vi "Gui.TopBar.Setting.vi"(7 "pane ref in":refnum<vi>, 8 "error in":errorcluster, 9 "values":T1={"OK"=FALSE, "Cancel"=FALSE, "Reload"=FALSE, "Save"=FALSE, "Module name"="NAME"}, 10 "visibility":T6, 11 "top bar ref in":refnum<vi>) -> (0 "error out":errorcluster, 3 "top bar ref out":refnum<vi>)   [LabVIEW 2019, in "Main.lvlib"]
uses:
  Main.lvlib
  Gui.TopBar.Visibility.ctl
  Gui.TopBar.ctl
  Framework/Tools/controls/buttons/OK.ctl
  Framework/Tools/controls/buttons/Cancel.ctl
  Framework/Tools/controls/buttons/Reload.ctl
  Framework/Tools/controls/buttons/Save.ctl
  Framework/Tools/Tools.lvlib
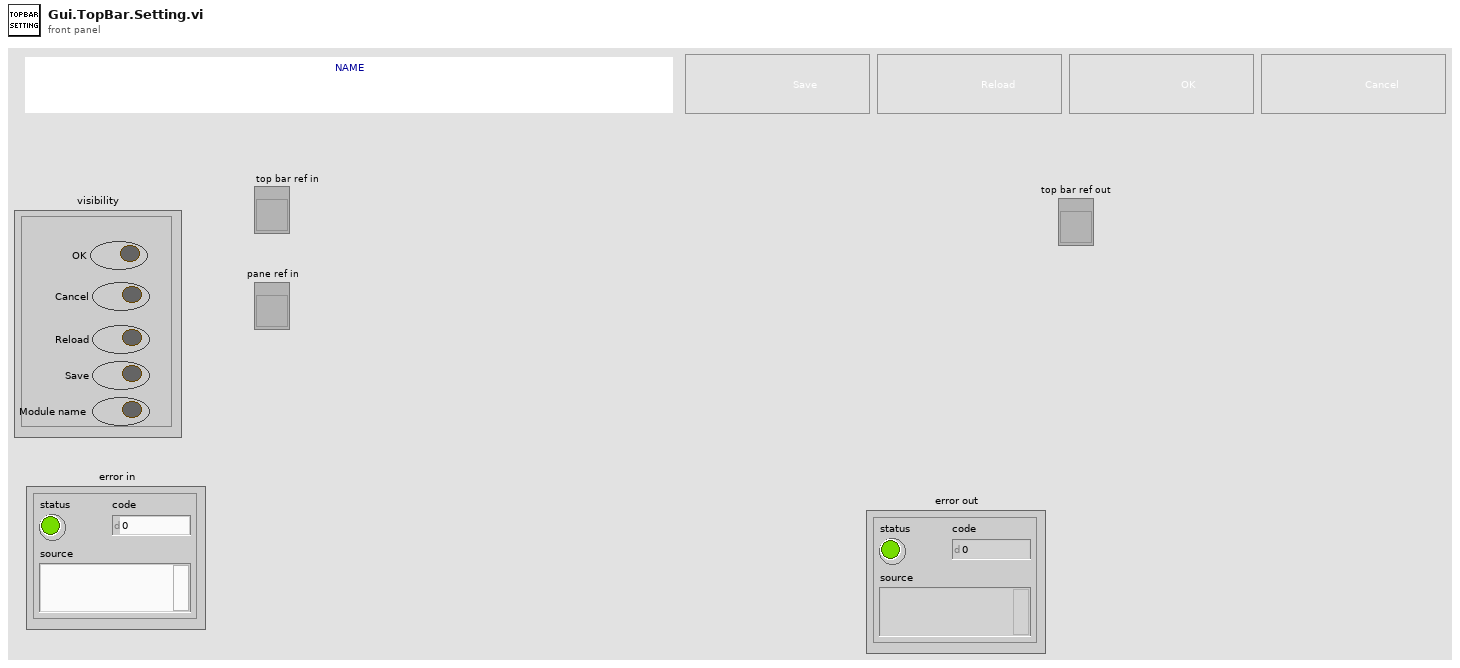
[diagram p1: front panel]
types:
  T1 = typedef "Main.lvlib/Gui.TopBar.ctl" = cluster{"OK":T2, "Cancel":T3, "Reload":T4, "Save":T5, "Module name":string}
  T2 = typedef "Tools.lvlib/OK.ctl" = bool
  T3 = typedef "Tools.lvlib/Cancel.ctl" = bool
  T4 = typedef "Tools.lvlib/Reload.ctl" = bool
  T5 = typedef "Tools.lvlib/Save.ctl" = bool
  T6 = typedef "Main.lvlib/Gui.TopBar.Visibility.ctl" = cluster{"OK":bool, "Cancel":bool, "Reload":bool, "Save":bool, "Module name":bool}
  T7 = typedef "LVPositionTypeDef.ctl" = cluster{"Left":i32, "Top":i32}
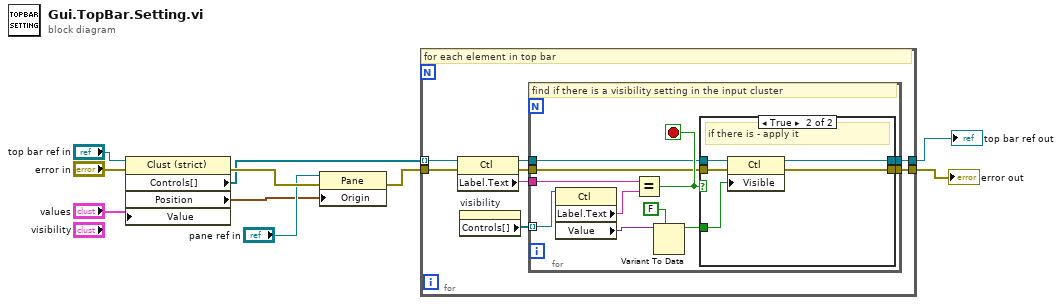
[diagram p0: block diagram]
diagram:
  n1 = property on="Property Node" class="Clust (strict)"(reference="top bar ref in", error in="error in", "Value"="values") -> (error out=w6:errorcluster, "Controls[]"=w2:refnum<vi>[], "Position"=w3:T7)  [unwired: 1 out]
  n2 = property on="Property Node" class="Pane"(reference="pane ref in", error in=w6, "Origin"=w3) -> (error out=w5:errorcluster)  [unwired: 1 out]
  n3 = for {
    tunnel: w2 -> [w18] mode=indexing
    tunnel: w5 -> [w13]
    tunnel: [w12] -> w8
    tunnel: [w11] -> w7
    # "for each element in top bar"
    n4 = property on="Property Node" class="Ctl"(reference=w18, error in=w13) -> (reference out=w15:refnum<vi>, error out=w14:errorcluster, "Label.Text"=w16:string)
    n5 = property on="visibility" class="Clust (strict)"() -> ("Controls[]"=w17:refnum<vi>[])  [unwired: 2 in, 2 out]
    n6 = for {
      tunnel: w17 -> [w29] mode=indexing
      tunnel: w16 -> [w28]
      tunnel: w15 -> [w25]
      tunnel: w14 -> [w21]
      tunnel: [w20] -> w12
      tunnel: [w19] -> w11
      stop <- w26 stop-if-true
      # "find if there is a visibility setting in the input cluster"
      n7 = property on="Property Node" class="Ctl"(reference=w29) -> ("Label.Text"=w27:string, "Value"=w24:variant)  [unwired: 1 in, 2 out]
      n8 = Equal?(x=w28, y=w27) -> (x = y?=w26:bool)
      n9 = Variant To Data(type=FALSE, Variant=w24) -> (data=w22:bool)  [unwired: 1 in, 1 out]
      n10 = case shown="True" w26 {
        tunnel: w25 -> [w30 w36]
        tunnel: w22 -> [_ w35]
        tunnel: w21 -> [w31 w34]
        tunnel: [w31 w33] -> w20
        tunnel: [w30 w32] -> w19
        frame False {
          # "if not, skip"
        }
        frame True {
          # "if there is - apply it"
          n11 = property on="Property Node" class="Ctl"(reference=w36, error in=w34, "Visible"=w35) -> (reference out=w32:refnum<vi>, error out=w33:errorcluster)
        }
      }
    }
  }
  "error out" <- w8
  "top bar ref out" <- w7
